vi "boolean_conversion_sub.vi"(11 "Array in":bool[](array[boolean])) -> (3 "Array out":u8[](array[numeric]))   [LabVIEW 2021]
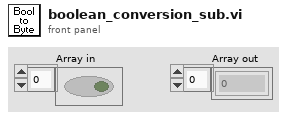
[diagram p1: front panel]
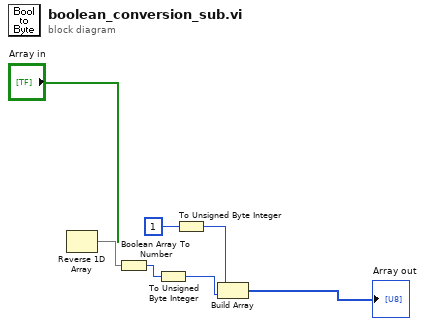
[diagram p0: block diagram]
diagram:
  n1 = Reverse 1D Array(array="Array in") -> (reversed array=w3:bool[])
  n2 = Boolean Array To Number(Boolean array=w3) -> (number=w1:u32)
  n3 = To Unsigned Byte Integer(number=w1) -> (unsigned 8bit integer=w7:u8)
  n4 = To Unsigned Byte Integer(number=u8 1) -> (unsigned 8bit integer=w6:u8)
  n5 = Build Array(w6, w7) -> (→"Array out":u8[])
